vi "Set Timestamp.vi"(8 "error in (no error)":errorcluster, 10 "Time Stamp":timestamp, 11 "JSON Scalar in":refnum<class "JSON Scalar.lvclass">) -> (0 "error out":errorcluster, 3 "JSON Scalar out":refnum<class "JSON Scalar.lvclass">)   [LabVIEW 2011, in "JSON Scalar.lvclass"]
doc: "Stores a <b>Time Stamp</b> as a <b>JSON Scalar</b>.\nUses the UTC formatter %Y-%m-%dT%H:%M:%S%3uZ\n\nCopyright 2012 James David Powell, Shaun Rumbell and Ton Plomp\nMore information on http://lavag.org/topic/16217-cr-json-labview"
uses:
  JSON Scalar.lvclass
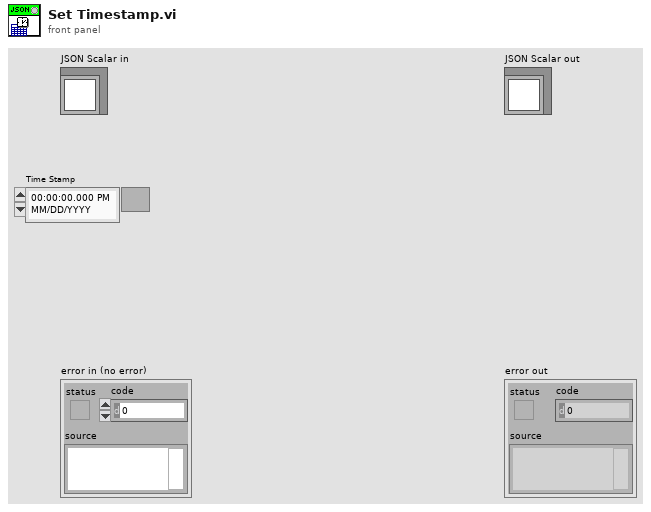
[diagram p1: front panel]
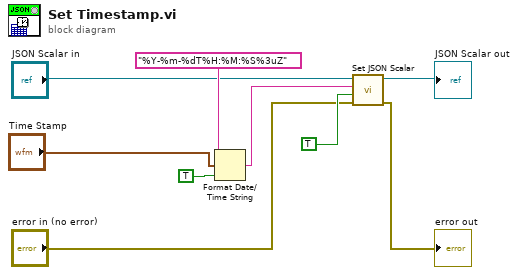
[diagram p0: block diagram]
diagram:
  n1 = Format Date/Time String(time format string (%c)="%Y-%m-%dT%H:%M:%S%3uZ", seconds (now)="Time Stamp", UTC format=TRUE) -> (date/time string=w8:string)
  n2 = call "Set JSON Scalar.vi"("error in (no error)"="error in (no error)", "Set as a JSON string (F)"=TRUE, "LabVIEW Text"=w8, "JSON Scalar in"="JSON Scalar in") -> ("error out"=→"error out":errorcluster, "JSON Scalar out"=→"JSON Scalar out":refnum<class "JSON Scalar.lvclass">)  [unwired: 6 in]
